vi "FaceDistance.vi"(8 "error in (no error)":errorcluster, 9 "faceToCompare":refnum<k24>, 10 "FaceEncoding":refnum<k24>, 11 "FaceRecognition in":refnum<class "FaceRecognition.lvclass">) -> (0 "error out":errorcluster, 2 "FaceDistance":dbl, 3 "FaceRecognition out":refnum<class "FaceRecognition.lvclass">)   [LabVIEW 2020, in "FaceRecognitionDotNet.lvlib" / "FaceRecognition.lvclass"]
uses:
  FaceRecognition.lvclass
  dll/FaceRecognitionDotNet.dll
  FaceRecognition.lvclass/FaceRecognition.ctl
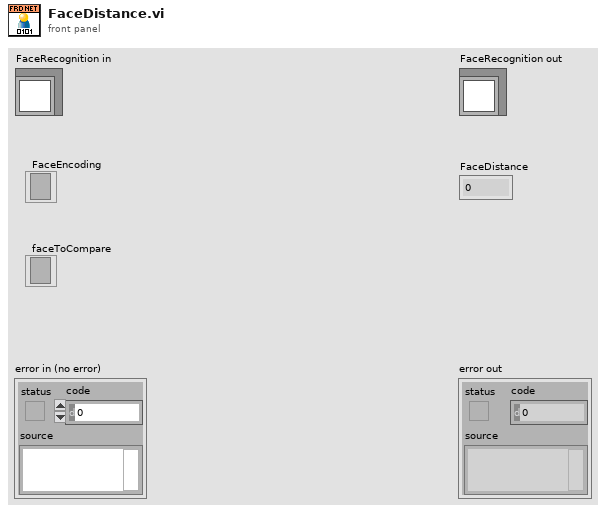
[diagram p1: front panel]
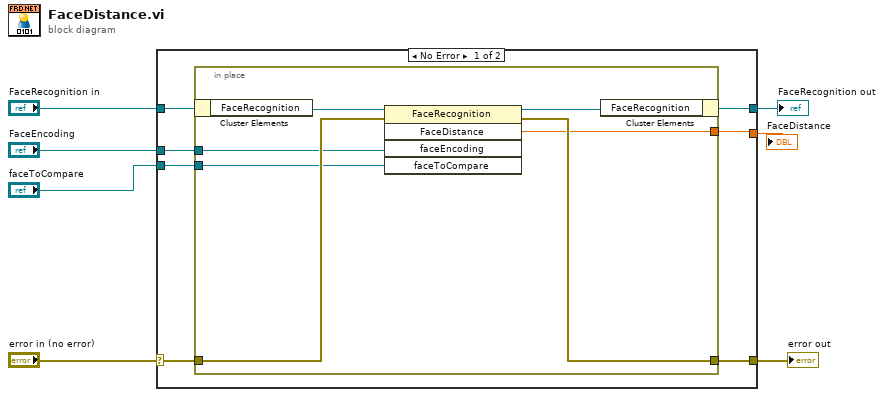
[diagram p0: block diagram]
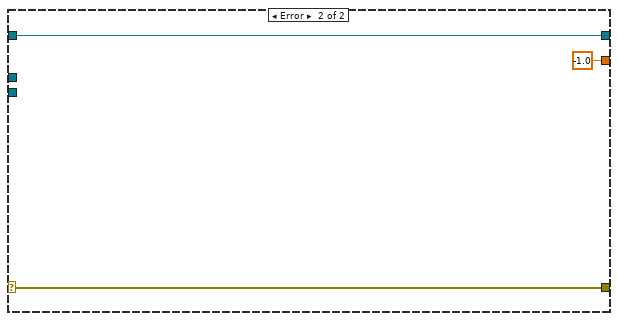
[diagram p2: hidden frame]
diagram:
  n1 = case shown="No Error" "error in (no error)" {
    selector: "error in (no error)" -> [w12 w24]
    tunnel: [w11 w24] -> w6
    tunnel: [w13 w23] -> w4
    tunnel: "FaceRecognition in" -> [w14 w23]
    tunnel: [w10 -1.0 ("FaceDistance")] -> w1
    tunnel: "FaceEncoding" -> [w9 _]
    tunnel: "faceToCompare" -> [w8 _]
    frame No Error {
      n2 = in-place {
        in-place-border: w12 -> [w19]
        in-place-border: [w18] -> w11
        in-place-border: [w17] -> w10
        in-place-border: w9 -> [w16]
        in-place-border: w8 -> [w15]
        n3 = in-place-cluster #1(w14) -> ("FaceRecognition"=w21:refnum<k24>)
        n4 = invoke class="FaceRecognition" method="FaceDistance"(reference=w21, error in=w19, "faceEncoding"=w16, "faceToCompare"=w15) -> (reference out=w20:refnum<k24>, error out=w18:errorcluster, "FaceDistance"=w17:dbl)  [unwired: 1 in, 2 out]
        n5 = in-place-cluster #1("FaceRecognition"=w20) -> (w13:refnum<class "FaceRecognition.lvclass">)
      }
    }
    frame Error {
    }
  }
  "error out" <- w6
  "FaceRecognition out" <- w4
  "FaceDistance" <- w1
